vi "All Tubes ON - OFF.vi"(6 "Tubes ON/OFF":bool, 7 "Number of tubes":i32=65, 11 "First Tube":i32) -> ()   [LabVIEW 2020]
uses:
  <vilib>/DAQmx/write.llb/DAQmx Write (Digital U8 1Chan 1Samp).vi
  <vilib>/DAQmx/create/channels.llb/DAQmx Create Channel (DO-Digital Output).vi
  <vilib>/DAQmx/miscellaneous.llb/DAQmx Fill In Error Info.vi
panel:
  in  "lines 2":tag="Dev2/port0/line0:7"
  out "Status(U8)":u8
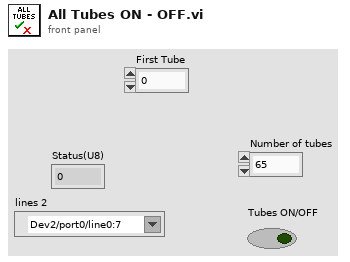
[diagram p1: front panel]
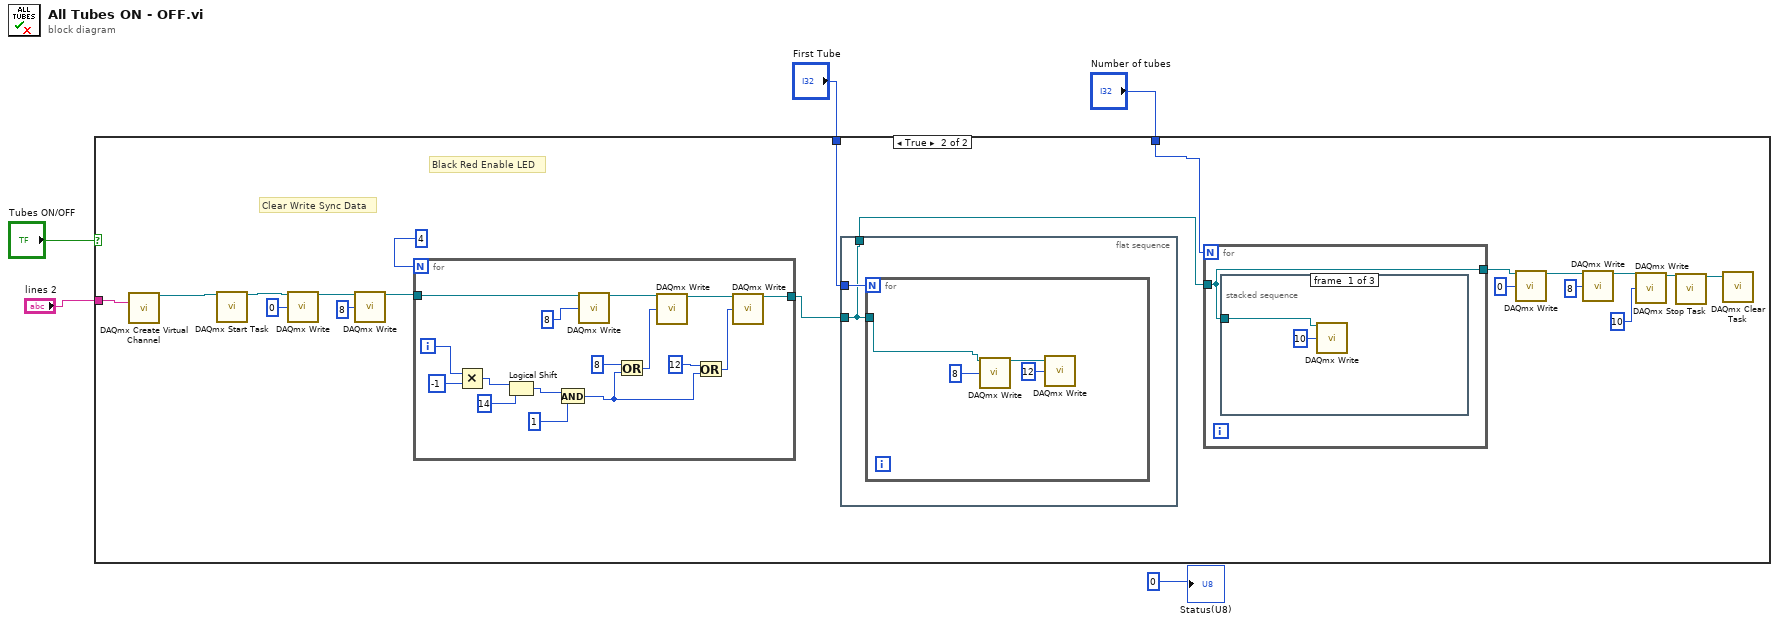
[diagram p0: block diagram]
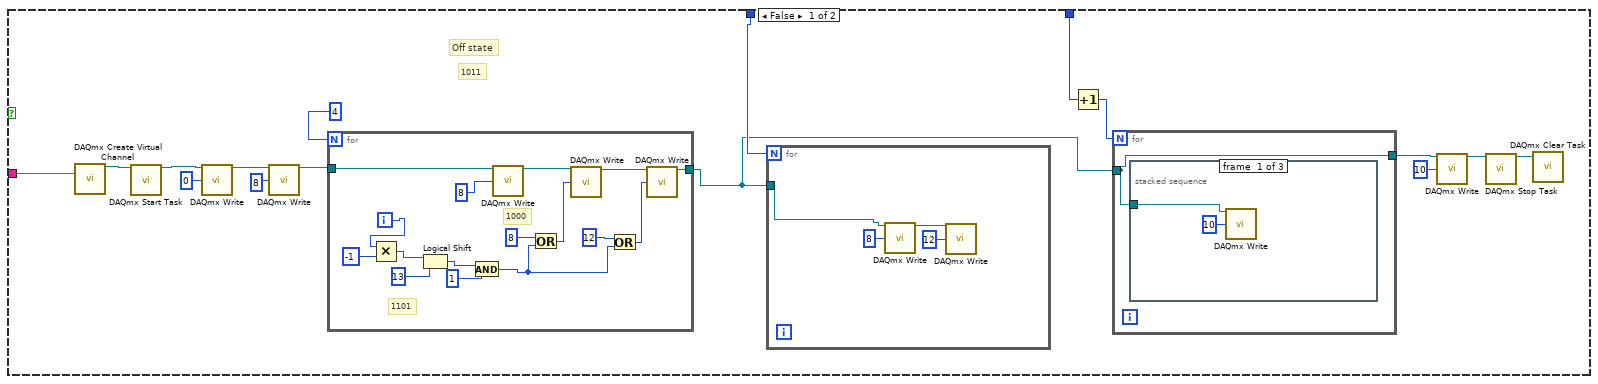
[diagram p2: hidden frame]
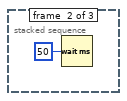
[diagram p3: hidden frame]
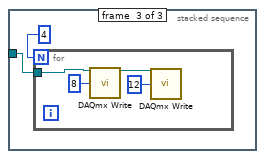
[diagram p4: hidden frame]
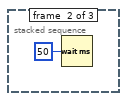
[diagram p5: hidden frame]
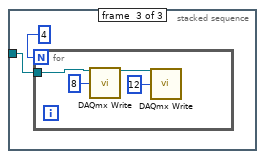
[diagram p6: hidden frame]
diagram:
  n1 = case shown="True" "Tubes ON/OFF" {
    tunnel: "Number of tubes" -> [w9 w59]
    tunnel: "lines 2" -> [w8 w63]
    tunnel: "First Tube" -> [w7 w62]
    frame False {
      # "Off state"
      # "1011"
      n2 = call-poly <vilib>:"DAQmx Create Virtual Channel.vi"("lines"=w8) -> ("task out"=w21:refnum<k21>)  [unwired: 13 in, 1 out]
      n3 = call <vilib>:"DAQmx Start Task.vi"("task/channels in"=w21) -> ("task out"=w14:refnum<k21>)  [unwired: 13 in, 1 out]
      n4 = call-poly <vilib>:"DAQmx Write.vi"("task/channels in"=w14, "data"=u8 0) -> ("task out"=w13:refnum<k21>)  [unwired: 11 in, 2 out]
      n5 = call-poly <vilib>:"DAQmx Write.vi"("task/channels in"=w13, "data"=u8 8) -> ("task out"=w18:refnum<k21>)  [unwired: 11 in, 2 out]
      n6 = for {
        N: 4 -> [_]
        tunnel: w18 -> [w40]
        tunnel: [w37] -> w6
        i -> [w49]
        # "1000"
        # "1101"
        n7 = Multiply(x=w49, y=-1) -> (x*y=w47:i32)
        n8 = Logical Shift(y=w47, x=u8 13) -> (x << y=w51:u8)
        n9 = And(x=w51, y=u32 1) -> (x .and. y?=w43:u32)
        n10 = call-poly <vilib>:"DAQmx Write.vi"("task/channels in"=w40, "data"=u32 8 ("x")) -> ("task out"=w39:refnum<k21>)  [unwired: 11 in, 2 out]
        n11 = Or(x=u32 8, y=w43) -> (x .or. y?=w44:u32)
        n12 = call-poly <vilib>:"DAQmx Write.vi"("task/channels in"=w39, "data"=w44) -> ("task out"=w38:refnum<k21>)  [unwired: 11 in, 2 out]
        n13 = Or(x=u32 12, y=w43) -> (x .or. y?=w41:u32)
        n14 = call-poly <vilib>:"DAQmx Write.vi"("task/channels in"=w38, "data"=w41) -> ("task out"=w37:refnum<k21>)  [unwired: 11 in, 2 out]
      }
      n15 = for {
        N: w7 -> [_]
        tunnel: w6 -> [w22]
        n16 = call-poly <vilib>:"DAQmx Write.vi"("task/channels in"=w22, "data"=u8 8) -> ("task out"=w23:refnum<k21>)  [unwired: 11 in, 2 out]
        n17 = call-poly <vilib>:"DAQmx Write.vi"("task/channels in"=w23, "data"=u8 12) -> ()  [unwired: 11 in, 3 out]
      }
      n18 = Increment(x=w9) -> (x+1=w10:i32)
      n19 = for {
        N: w10 -> [_]
        tunnel: w6 -> [w26]
        tunnel: [w26] -> w11
        n20 = stacked-sequence {
          tunnel: w26 -> [w27 _ w30]
          frame #0 {
            n21 = call-poly <vilib>:"DAQmx Write.vi"("task/channels in"=w27, "data"=u8 10) -> ()  [unwired: 11 in, 3 out]
          }
          frame #1 {
            n22 = Wait (ms)(milliseconds to wait=u32 50) -> ()  [unwired: 1 out]
          }
          frame #2 {
            n23 = for {
              N: 4 -> [_]
              tunnel: w30 -> [w33]
              n24 = call-poly <vilib>:"DAQmx Write.vi"("task/channels in"=w33, "data"=u8 8) -> ("task out"=w32:refnum<k21>)  [unwired: 11 in, 2 out]
              n25 = call-poly <vilib>:"DAQmx Write.vi"("task/channels in"=w32, "data"=u8 12) -> ()  [unwired: 11 in, 3 out]
            }
          }
        }
      }
      n26 = call-poly <vilib>:"DAQmx Write.vi"("task/channels in"=w11, "data"=u8 10) -> ("task out"=w17:refnum<k21>)  [unwired: 11 in, 2 out]
      n27 = call <vilib>:"DAQmx Stop Task.vi"("task/channels in"=w17) -> ("task out"=w20:refnum<k21>)  [unwired: 13 in, 1 out]
      n28 = call <vilib>:"DAQmx Clear Task.vi"("task in"=w20) -> ()  [unwired: 14 in, 1 out]
    }
    frame True {
      # "Black Red Enable LED"
      # "Clear Write Sync Data"
      n29 = call-poly <vilib>:"DAQmx Create Virtual Channel.vi"("lines"=w63) -> ("task out"=w71:refnum<k21>)  [unwired: 13 in, 1 out]
      n30 = call <vilib>:"DAQmx Start Task.vi"("task/channels in"=w71) -> ("task out"=w66:refnum<k21>)  [unwired: 13 in, 1 out]
      n31 = call-poly <vilib>:"DAQmx Write.vi"("task/channels in"=w66, "data"=u8 0) -> ("task out"=w65:refnum<k21>)  [unwired: 11 in, 2 out]
      n32 = call-poly <vilib>:"DAQmx Write.vi"("task/channels in"=w65, "data"=u8 8) -> ("task out"=w68:refnum<k21>)  [unwired: 11 in, 2 out]
      n33 = for {
        N: 4 -> [_]
        tunnel: w68 -> [w92]
        tunnel: [w89] -> w61
        i -> [w101]
        n34 = Multiply(x=w101, y=-1) -> (x*y=w99:i32)
        n35 = Logical Shift(y=w99, x=u8 14) -> (x << y=w103:u8)
        n36 = And(x=w103, y=u32 1) -> (x .and. y?=w95:u32)
        n37 = call-poly <vilib>:"DAQmx Write.vi"("task/channels in"=w92, "data"=u32 8 ("x")) -> ("task out"=w91:refnum<k21>)  [unwired: 11 in, 2 out]
        n38 = Or(x=u32 8, y=w95) -> (x .or. y?=w96:u32)
        n39 = call-poly <vilib>:"DAQmx Write.vi"("task/channels in"=w91, "data"=w96) -> ("task out"=w90:refnum<k21>)  [unwired: 11 in, 2 out]
        n40 = Or(x=u32 12, y=w95) -> (x .or. y?=w93:u32)
        n41 = call-poly <vilib>:"DAQmx Write.vi"("task/channels in"=w90, "data"=w93) -> ("task out"=w89:refnum<k21>)  [unwired: 11 in, 2 out]
      }
      n42 = flat-sequence {
        tunnel: w62 -> [w73]
        tunnel: w61 -> [w72]
        tunnel: [w72] -> w60
        frame #0 {
          n43 = for {
            N: w73 -> [_]
            tunnel: w72 -> [w74]
            n44 = call-poly <vilib>:"DAQmx Write.vi"("task/channels in"=w74, "data"=u8 8) -> ("task out"=w75:refnum<k21>)  [unwired: 11 in, 2 out]
            n45 = call-poly <vilib>:"DAQmx Write.vi"("task/channels in"=w75, "data"=u8 12) -> ()  [unwired: 11 in, 3 out]
          }
        }
      }
      n46 = for {
        N: w59 -> [_]
        tunnel: w60 -> [w78]
        tunnel: [w78] -> w55
        n47 = stacked-sequence {
          tunnel: w78 -> [w79 _ w82]
          frame #0 {
            n48 = call-poly <vilib>:"DAQmx Write.vi"("task/channels in"=w79, "data"=u8 10) -> ()  [unwired: 11 in, 3 out]
          }
          frame #1 {
            n49 = Wait (ms)(milliseconds to wait=u32 50) -> ()  [unwired: 1 out]
          }
          frame #2 {
            n50 = for {
              N: 4 -> [_]
              tunnel: w82 -> [w85]
              n51 = call-poly <vilib>:"DAQmx Write.vi"("task/channels in"=w85, "data"=u8 8) -> ("task out"=w84:refnum<k21>)  [unwired: 11 in, 2 out]
              n52 = call-poly <vilib>:"DAQmx Write.vi"("task/channels in"=w84, "data"=u8 12) -> ()  [unwired: 11 in, 3 out]
            }
          }
        }
      }
      n53 = call-poly <vilib>:"DAQmx Write.vi"("task/channels in"=w55, "data"=u8 0) -> ("task out"=w56:refnum<k21>)  [unwired: 11 in, 2 out]
      n54 = call-poly <vilib>:"DAQmx Write.vi"("task/channels in"=w56, "data"=u8 8) -> ("task out"=w54:refnum<k21>)  [unwired: 11 in, 2 out]
      n55 = call-poly <vilib>:"DAQmx Write.vi"("task/channels in"=w54, "data"=u8 10) -> ("task out"=w53:refnum<k21>)  [unwired: 11 in, 2 out]
      n56 = call <vilib>:"DAQmx Stop Task.vi"("task/channels in"=w53) -> ("task out"=w70:refnum<k21>)  [unwired: 13 in, 1 out]
      n57 = call <vilib>:"DAQmx Clear Task.vi"("task in"=w70) -> ()  [unwired: 14 in, 1 out]
    }
  }
  "Status(U8)" <- u8 0
